vi "TimeDelay.vi"(1 "Delay time (s)":dbl) -> (0 "Canceled":bool)   [LabVIEW 2021]
uses:
  Globals and TypeDefs/Global Varibal Control.vi
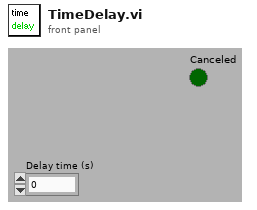
[diagram p1: front panel]
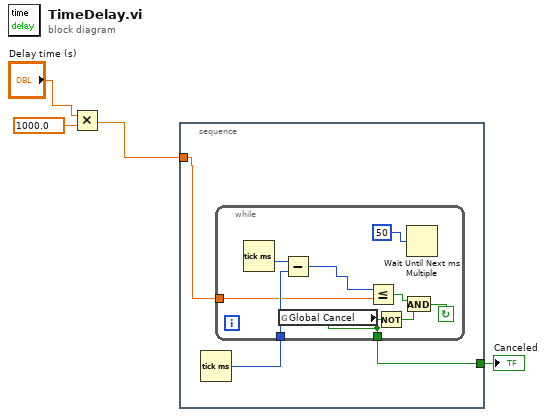
[diagram p0: block diagram]
diagram:
  n1 = Multiply(x="Delay time (s)", y=1000.0) -> (x*y=w3:dbl)
  n2 = stacked-sequence {
    tunnel: [w6] -> w2
    tunnel: w3 -> [w5]
    frame #0 {
      n3 = Tick Count (ms)() -> (millisecond timer value=w7:u32)
      n4 = while {
        tunnel: [w8] -> w6
        tunnel: w5 -> [w13]
        tunnel: w7 -> [w15]
        stop <- w10 continue-if-true
        n5 = Tick Count (ms)() -> (millisecond timer value=w16:u32)
        n6 = global read "Global Varibal Control.vi" "Global Cancel"() -> (w8:bool)
        n7 = Subtract(x=w16, y=w15) -> (x-y=w9:u32)
        n8 = Less Or Equal?(x=w9, y=w13) -> (x <= y?=w11:bool)
        n9 = Not(x=w8) -> (.not. x?=w12:bool)
        n10 = And(x=w11, y=w12) -> (x .and. y?=w10:bool)
        n11 = Wait Until Next ms Multiple(millisecond multiple=u32 50) -> ()  [unwired: 1 out]
      }
    }
  }
  "Canceled" <- w2
